vi "Telnet_RW_wResp_v2 - Copy.vi"() -> ()   [LabVIEW 2018]
panel:
  out "offset past match":i32
  out "match substring":string
  in  "regular expression":string="->"
  in  "string":string
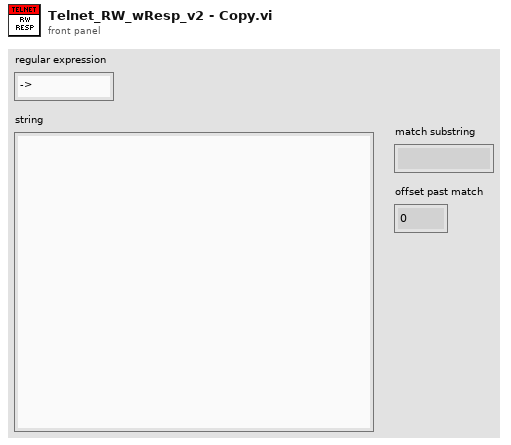
[diagram p1: front panel]
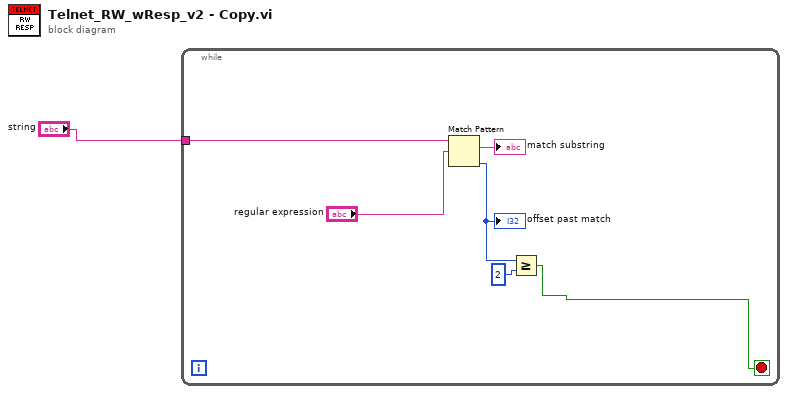
[diagram p0: block diagram]
diagram:
  n1 = while {
    tunnel: "string" -> [w2]
    stop <- w3 stop-if-true
    n2 = Match Pattern(string=w2, regular expression="regular expression") -> (match substring=→"match substring":string, offset past match=w5:i32)  [unwired: 1 in, 2 out]
    "offset past match" <- w5
    n3 = Greater Or Equal?(x=w5, y=2) -> (x >= y?=w3:bool)
  }
